vi "LFA_Close.vi"(8 "error in (no error)":errorcluster, 11 "LightField Automation in":refnum<class "LightField Automation.lvclass">) -> (0 "error out":errorcluster, 3 "LightField Automation out":refnum<class "LightField Automation.lvclass">)   [LabVIEW 2013, in "LightField Automation.lvclass"]
uses:
  LightField Automation.lvclass
  LightField Automation.lvclass/LightField Automation.ctl
  C:/Program Files/Princeton Instruments/LightField/PrincetonInstruments.LightField.AutomationV3.dll
  Program Files/Princeton Instruments/LightField/PrincetonInstruments.LightField.AutomationV3.dll
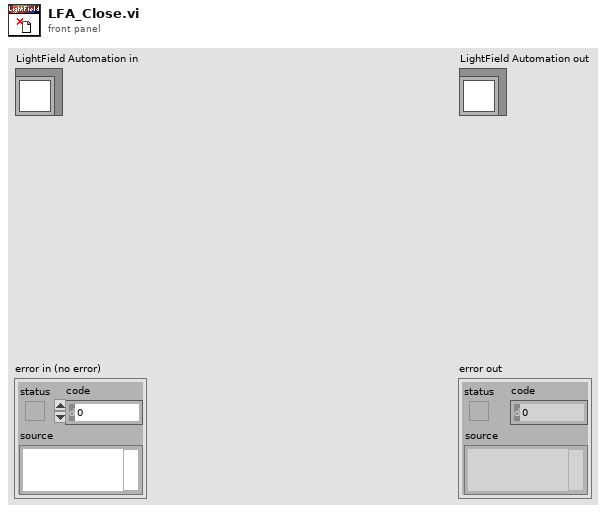
[diagram p1: front panel]
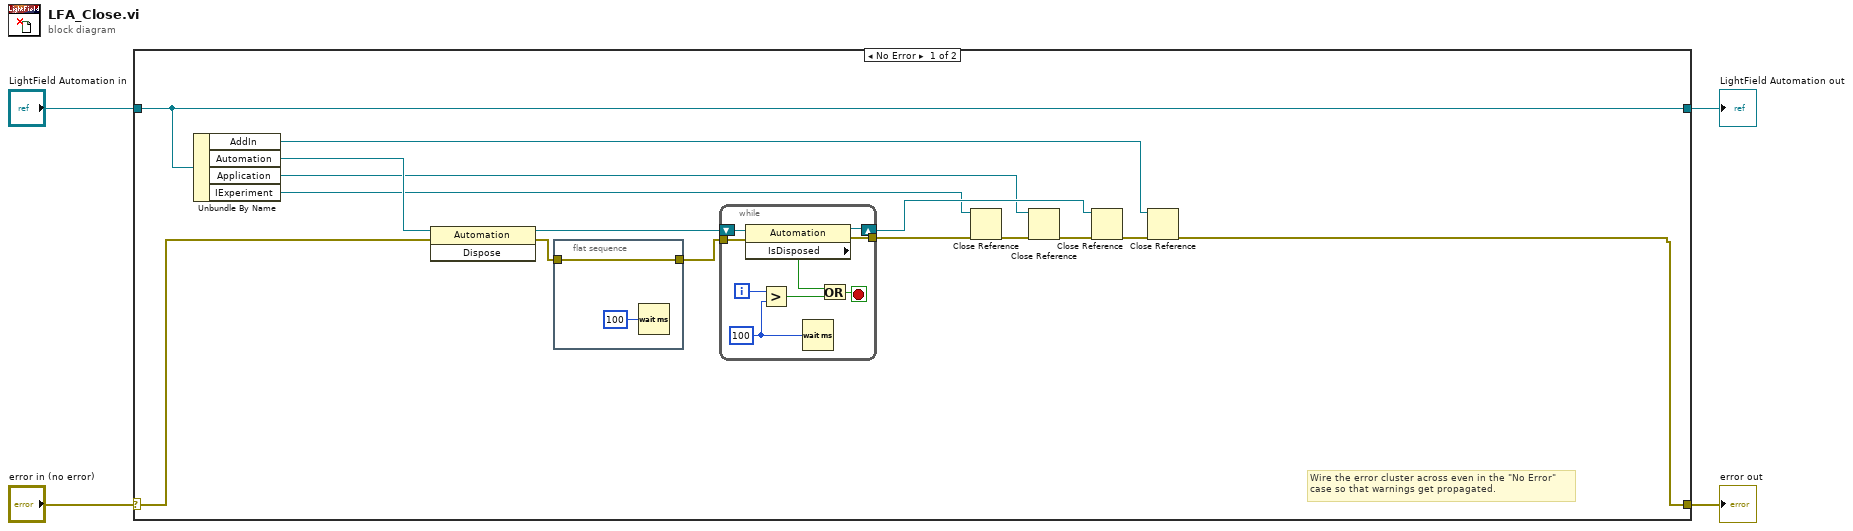
[diagram p0: block diagram]
diagram:
  n1 = case shown="No Error" "error in (no error)" {
    selector: "error in (no error)" -> [w18 w32]
    tunnel: [w6 w32] -> w3
    tunnel: [w5 w31] -> w1
    tunnel: "LightField Automation in" -> [w5 w31]
    frame No Error {
      # "Wire the error cluster across even in the \"No Error\"\ncase so that warnings get propagated."
      n2 = Unbundle By Name(w5) -> ("AddIn"=w9:refnum<k24>, "Automation"=w19:refnum<k24>, "Application"=w8:refnum<k24>, "IExperiment"=w7:refnum<k24>)
      n3 = invoke class="Automation" method="Dispose"(reference=w19, error in=w18) -> (reference out=w15:refnum<k24>, error out=w17:errorcluster)  [unwired: 1 in, 1 out]
      n4 = flat-sequence {
        tunnel: w17 -> [w21]
        tunnel: [w21] -> w16
        frame #0 {
          n5 = Wait (ms)(milliseconds to wait=u32 100) -> ()  [unwired: 1 out]
        }
      }
      n6 = while {
        tunnel: w16 -> [w29]
        shift-right: [w28] -> w10
        shift-left: w15 -> [w30]
        tunnel: [w27] -> w14
        i -> [w26]
        stop <- w24 stop-if-true
        w25 = u32 100 ("milliseconds to wait")
        n7 = property class="Automation"(reference=w30, error in=w29) -> (reference out=w28:refnum<k24>, error out=w27:errorcluster, "IsDisposed"=w22:bool)
        n8 = Greater?(x=w26, y=w25) -> (0:w23:bool)
        n9 = Wait (ms)(milliseconds to wait=w25) -> ()  [unwired: 1 out]
        n10 = Or(x=w22, y=w23) -> (x .or. y?=w24:bool)
      }
      n11 = Close Reference(reference=w7, error in (no error)=w14) -> (error out=w13:errorcluster)
      n12 = Close Reference(reference=w8, error in (no error)=w13) -> (error out=w12:errorcluster)
      n13 = Close Reference(reference=w10, error in (no error)=w12) -> (error out=w11:errorcluster)
      n14 = Close Reference(reference=w9, error in (no error)=w11) -> (error out=w6:errorcluster)
    }
    frame Error {
    }
  }
  "error out" <- w3
  "LightField Automation out" <- w1
